vi "UDP3GLOB.vi"() -> ()   [LabVIEW 2009]
uses:
  UDP 3.ctl
panel:
  in  "stop":bool
  in  "UDP 3":T1
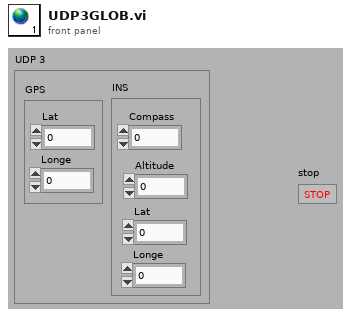
[diagram p1: front panel]
types:
  T1 = typedef "UDP 3.ctl" = cluster{"GPS":cluster{"Lat":dbl, "Longe":dbl}, "INS":cluster{"Compass":dbl, "Altitude":dbl, "Lat":dbl, "Longe":dbl}}
diagram:
